vi "Get Data Channel Property.vi"(8 "error in (no error)":errorcluster, 11 "Item Ref in":T1 format="%.0x") -> (0 "error out":errorcluster, 2 "Data Channel Property":T2={"pkid"=0, "Signalname"="", "PlayerID"=1, "WheelID"=0}, 3 "Item Ref out":T1 format="%.0x")   [LabVIEW 2023]
uses:
  <vilib>/NI VeriStand/Custom Device API/Custom Device Item Ref.ctl
  Data Channel Custom Property.ctl
  <vilib>/NI VeriStand/Custom Device API/Get Item Property (Variant).vi
  <vilib>/NI VeriStand/Custom Device API/Custom Device API.lvlib
  Vires VTD System Explorer.lvlib
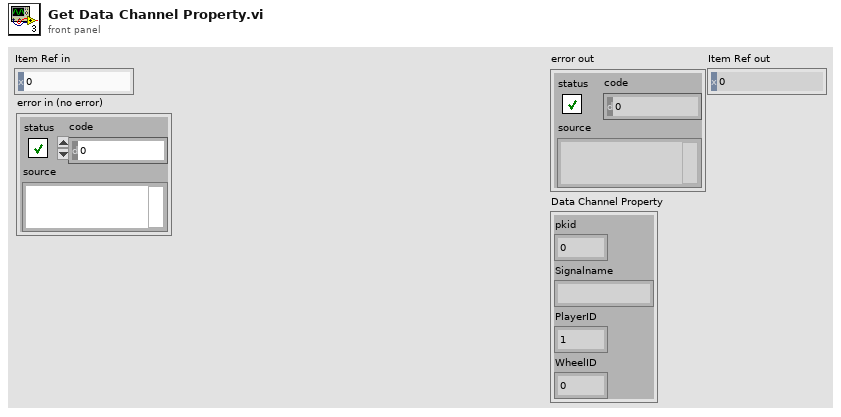
[diagram p1: front panel]
types:
  T1 = typedef "Custom Device API.lvlib/Custom Device Item Ref.ctl" = u64
  T2 = typedef "Vires VTD System Explorer.lvlib/Data Channel Custom Property.ctl" = cluster{"pkid":u32, "Signalname":string, "PlayerID":u8, "WheelID":i32}
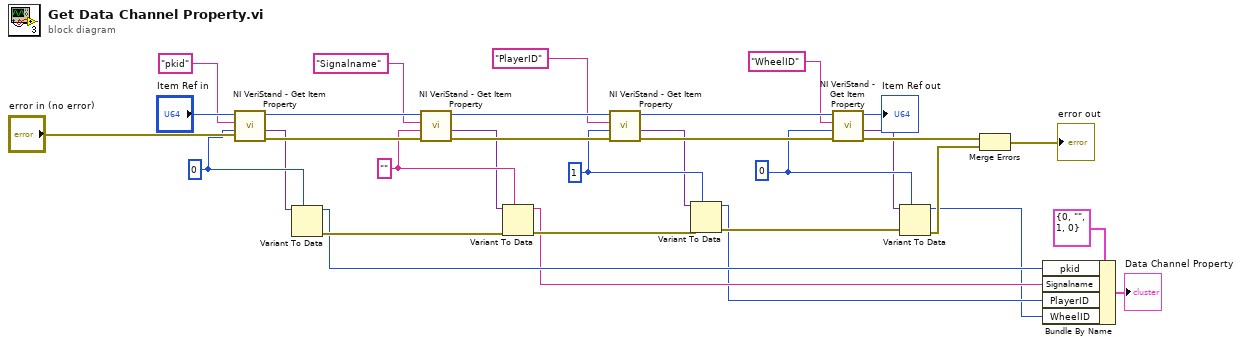
[diagram p0: block diagram]
diagram:
  w12 = 0 ("WheelID")
  w13 = u8 1 ("PlayerID")
  w14 = "" ("RDB Signalname")
  w15 = u32 0 ("Identifier")
  n1 = call-poly <vilib>:"NI VeriStand - Get Item Property.vi"("error in (no error)"="error in (no error)", "Default Value"=w15, "Property Name"="pkid" ("String"), "Item Ref in"="Item Ref in") -> ("error out"=w31:errorcluster, "Value"=w11:variant, "Item Ref out"=w32:T1)  [unwired: 4 in, 1 out]
  n2 = Variant To Data(type=w15, Variant=w11) -> (data=w6:u32, error out=w19:errorcluster)  [unwired: 1 in]
  n3 = call-poly <vilib>:"NI VeriStand - Get Item Property.vi"("error in (no error)"=w31, "Default Value"=w14, "Property Name"="Signalname" ("String"), "Item Ref in"=w32) -> ("error out"=w29:errorcluster, "Value"=w10:variant, "Item Ref out"=w30:T1)  [unwired: 4 in, 1 out]
  n4 = Variant To Data(error in=w19, type=w14, Variant=w10) -> (data=w5:string, error out=w18:errorcluster)
  n5 = call-poly <vilib>:"NI VeriStand - Get Item Property.vi"("error in (no error)"=w29, "Default Value"=w13, "Property Name"="PlayerID" ("String"), "Item Ref in"=w30) -> ("error out"=w27:errorcluster, "Value"=w9:variant, "Item Ref out"=w28:T1)  [unwired: 4 in, 1 out]
  n6 = Variant To Data(error in=w18, type=w13, Variant=w9) -> (data=w4:u8, error out=w17:errorcluster)
  n7 = call-poly <vilib>:"NI VeriStand - Get Item Property.vi"("error in (no error)"=w27, "Default Value"=w12, "Property Name"="WheelID" ("String"), "Item Ref in"=w28) -> ("error out"=w21:errorcluster, "Value"=w8:variant, "Item Ref out"=→"Item Ref out":T1)  [unwired: 4 in, 1 out]
  n8 = Variant To Data(error in=w17, type=w12, Variant=w8) -> (data=w3:i32, error out=w16:errorcluster)
  n9 = Merge Errors(w21, w16) -> (→"error out":errorcluster)
  n10 = Bundle By Name(cluster=T2 {"pkid"=0, "Signalname"="", "PlayerID"=1, "WheelID"=0} ("Data Channel Property"), "pkid"=w6, "Signalname"=w5, "PlayerID"=w4, "WheelID"=w3) -> (→"Data Channel Property":T2)
